vi "Send_command_and_check_response_number.vi"(5 "output cluster":T1 {"TimeStamp" format="%.2f"}, 6 "error in (no error)":errorcluster, 7 "Command":string="TIME", 8 "Set value":dbl format="%#_13g", 9 "TimeOut Time (s)":dbl=30.0 format="%#_13g") -> (0 "error IO":errorcluster, 1 "Return value":string)   [LabVIEW 2020]
uses:
  DataSocketCluster external.ctl
  vi Mode external.ctl
  04bf3837-9317-4129-9531-d6752085829f.vi
  <vilib>/Utility/error.llb/Error Cluster From Error Code.vi
  <vilib>/ErrorRing/Error Ring.xnode
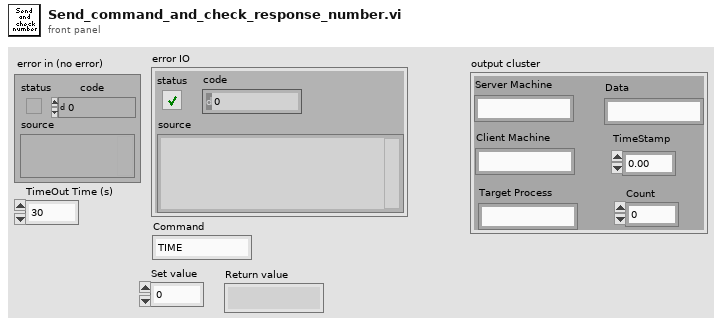
[diagram p1: front panel]
types:
  T1 = typedef "DataSocketCluster external.ctl" = cluster{"Server Machine":string, "Client Machine":string, "Data":string, "TimeStamp":dbl, "Count":i32, "Target Process":string}
  T2 = typedef "vi Mode external.ctl" = enum16{"Client", "Server"}
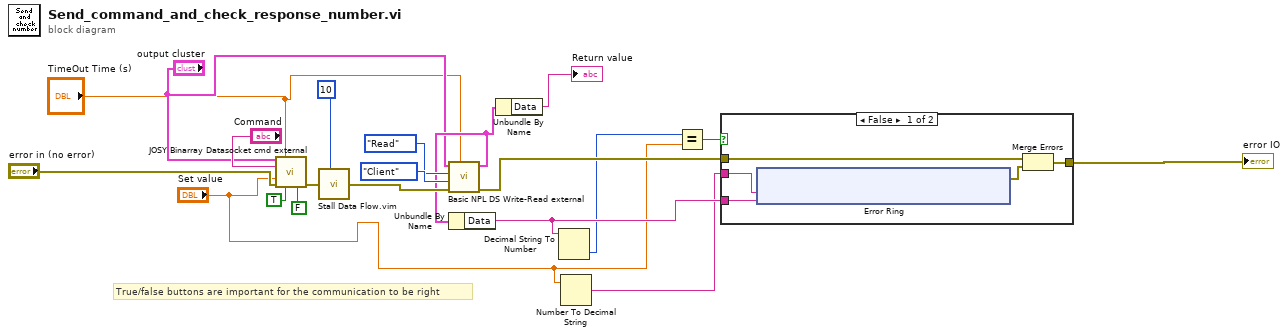
[diagram p0: block diagram]
diagram:
  # "True/false buttons are important for the communication to be right"
  n1 = call "JOSY Binarray Datasocket cmd external.vi"("DataSocketCluster In"="output cluster", "TimeOut Time (s)"="TimeOut Time (s)", "Command"="Command", "Value"="Set value", "error in (no error)"="error in (no error)", "Command has variable"=TRUE, "String"=FALSE) -> ("error out"=w17:errorcluster)  [unwired: 5 in, 3 out]
  n2 = call "Stall Data Flow.vim"("value in"=w17, "milliseconds to wait"=u32 10) -> ("value out"=w16:errorcluster)  [unwired: 1 out]
  n3 = call "Basic NPL DS Write-Read external.vi"("TimeOut Time (s)"="TimeOut Time (s)", "error in (no error)"=w16, "Server Mode"=vi_Mode_external."Client", "Operation Mode"=enum16{"Read", "Write", "Write/Read"}."Read", "DataSocketCluster In"="output cluster") -> ("error out"=w10:errorcluster, "DataSocketCluster Out"=w3:T1)  [unwired: 2 in, 1 out]
  n4 = Unbundle By Name(w3) -> ("Data"=w7:string)
  n5 = Unbundle By Name(w3) -> ("Data"=→"Return value":string)
  n6 = Decimal String To Number(string=w7) -> (number=w5:i32)  [unwired: 2 in, 1 out]
  n7 = Number To Decimal String(number="Set value") -> (decimal integer string=w6:string)  [unwired: 1 in]
  n8 = Equal?(x=w5, y="Set value") -> (x = y?=w12:bool)
  n9 = case shown="False" w12 {
    tunnel: w10 -> [w22 w34]
    tunnel: w6 -> [w25 _]
    tunnel: w7 -> [w24 _]
    tunnel: [w21 w34] -> w11
    frame False {
      n10 = xnode "Error Ring"("parameter 0"=w25, "parameter 1"=w24) -> ("error out"=w23:errorcluster)
      n11 = Merge Errors(w22, w23) -> (w21:errorcluster)
    }
    frame True {
    }
  }
  "error IO" <- w11
